vi "bulge wall align v0.2.vi"(8 "Error In":errorcluster) -> (0 "Error Out":errorcluster)   [LabVIEW 2019]
uses:
  <vilib>/platform/TimedLoop/XDataNode/XDataNode.xnode
  <vilib>/Platform/TimedLoop/XDataNode/nitl_modes.ctl
  <vilib>/Platform/TimedLoop/XDataNode/XDNodeRunTimeDep.lvlib
  <vilib>/Platform/TimedLoop/XDataNode/wakeup.ctl
  <vilib>/Platform/TimedLoop/XDataNode/timing_clust.ctl
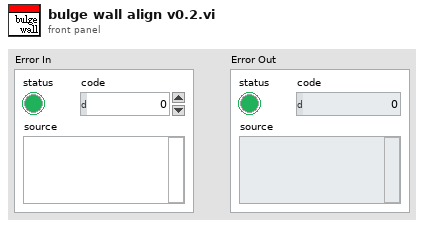
[diagram p1: front panel]
types:
  T1 = typedef "XDNodeRunTimeDep.lvlib/timing_clust.ctl" = cluster{"Expected End [f-1]":u64, "Actual End [f-1]":u64, "Finished Late? [f-1]":bool, "Expected End [i-1]":u64, "Actual End [i-1]":u64, "Finished Late? [i-1]":bool, "Expected Start [i]":u64, "Actual Start [i]":u64, "Expected Start [f]":u64, "Actual Start [f]":u64, "Source Name":string, "Structure Name":string, "Period":i64, "Deadline":i64, "Offset":i64, "Start":i64, "Priority":i32, "Timeout":i32, "Mode":T2, "Wakeup Reason":T3, "Error":errorcluster, "Source Type":string, "Secondary Source Type":string, "Global End Time":u64, "Global Start Time":u64, "Frame Duration":u64, "Iteration Duration":u64, "Assigned CPU":i32, "I/O Scan Engine Mode":u32}
  T2 = typedef "XDNodeRunTimeDep.lvlib/nitl_modes.ctl" = enum32{"No Change", "Process missed periods, maintain original phase", "Discard missed periods, maintain original phase", "Process missed periods, ignore original phase", "Discard missed periods, ignore original phase"}
  T3 = typedef "XDNodeRunTimeDep.lvlib/wakeup.ctl" = enum32{"Normal", "Aborted", "Asynchronous wakeup", "Timing source error", "Timed loop error", "Timeout"}
  T4 = typedef "IR out.ctl" = cluster{"DC estimate (V) 2":dbl, "DC estimate (V)":dbl, "AC estimate (Vrms)":dbl, "AC estimate (Vrms) 2":dbl}
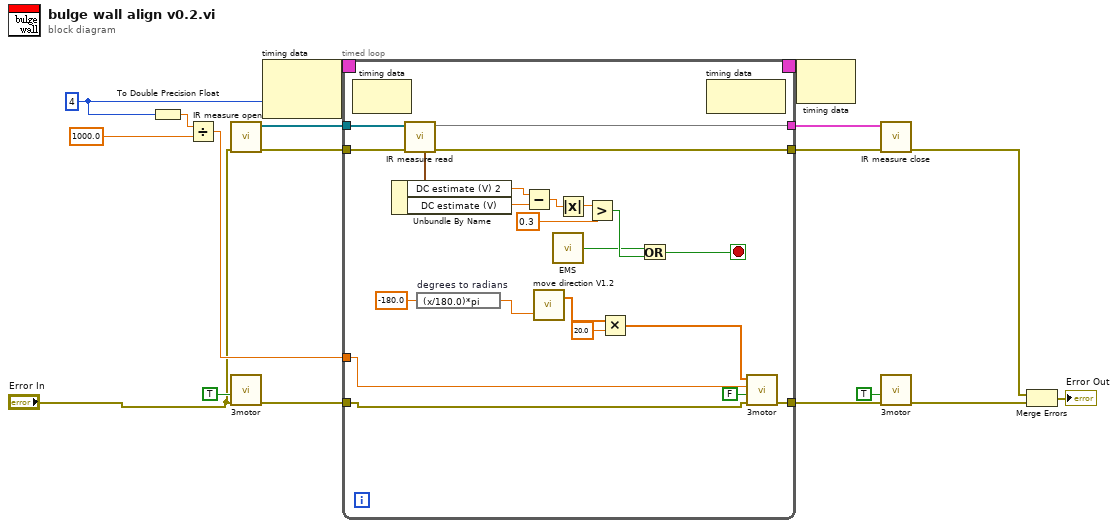
[diagram p0: block diagram]
diagram:
  w10 = i64 4 ("Period")
  n1 = To Double Precision Float(number=w10) -> (double precision float=w9:dbl)
  n2 = Divide(x=w9, y=1000.0) -> (x/y=w7:dbl)
  n3 = call "IR measure open.vi"("error in (no error)"="Error In") -> ("error out"=w15:errorcluster, "ref array"=w16:refnum<class "IR sensor.lvclass">[])  [unwired: 9 in]
  n4 = call "3motor.vi"("error in (no error)"="Error In", "Reset"=TRUE) -> ("error out"=w12:errorcluster)  [unwired: 9 in]
  n5 = node-c288(w10) -> (w18:T1)  [unwired: 1 in]
  n6 = timed-loop {
    timing: w18 -> [_]
    timing-out: [_] -> w17
    tunnel: w16 -> [w40]
    tunnel: w15 -> [w39]
    tunnel: [w38] -> w14
    tunnel: [w37] -> w13
    tunnel: w12 -> [w34]
    tunnel: [w36] -> w11
    tunnel: w7 -> [w33]
    stop <- w20 stop-if-true
    n7 = node-c288() -> ()  [unwired: 1 in, 1 out]
    n8 = call "IR measure read.vi"("error in (no error)"=w39, "ref array"=w40) -> ("error out"=w38:errorcluster, 3:w37, "output cluster"=w27:T4)  [unwired: 6 in, 1 out]
    n9 = Unbundle By Name(w27) -> ("DC estimate (V) 2"=w26:dbl, "DC estimate (V)"=w25:dbl)
    n10 = expression code="(x/180.0)*pi" "degrees to radians"(-180.0) -> (w31:dbl)
    n11 = Subtract(x=w26, y=w25) -> (x-y=w24:dbl)
    n12 = call "move direction V1.2.vi"("theta"=w31) -> ("out array"=w30:dbl[])  [unwired: 1 in, 1 out]
    n13 = call "EMS.vi"() -> ("A/DIO4 (Pin 19)"=w19:bool)
    n14 = Absolute Value(x=w24) -> (abs(x)=w23:dbl)
    n15 = Greater?(x=w23, y=0.3) -> (0:w21:bool)
    n16 = Multiply(x=w30, y=20.0) -> (x*y=w28:dbl[])
    n17 = Or(x=w19, y=w21) -> (x .or. y?=w20:bool)
    n18 = node-c288() -> ()  [unwired: 1 in, 1 out]
    n19 = call "3motor.vi"("error in (no error)"=w34, "Reset"=FALSE, "dt(s)"=w33, "Motor speed"=w28) -> ("error out"=w36:errorcluster)  [unwired: 7 in]
  }
  n20 = node-c288(w17) -> ()  [unwired: 1 out]
  n21 = call "IR measure close.vi"("error in (no error)"=w14, "AI Ref In"=w13) -> ("error out"=w3:errorcluster)  [unwired: 9 in]
  n22 = call "3motor.vi"("error in (no error)"=w11, "Reset"=TRUE) -> ("error out"=w4:errorcluster)  [unwired: 9 in]
  n23 = Merge Errors(w3, w4) -> (→"Error Out":errorcluster)
